vi "FGV_DataPackerQueueMetrics.vi"(7 "Enum":T1, 8 "Queue Size":i32, 9 "Elements bundled for serialisation":i32, 10 "# elements in queue":i32, 11 "Unique Banks to serialise":i32) -> (0 "Queue Size":i32, 1 "Elements bundled for serialisation":i32, 2 "# elements in queue":i32, 3 "Unique Banks to serialise":i32)   [LabVIEW 2018, in "feGEM DataPacker.lvlib"]
uses:
  Set_And_Get_Enum.ctl
  feGEM DataPacker.lvlib
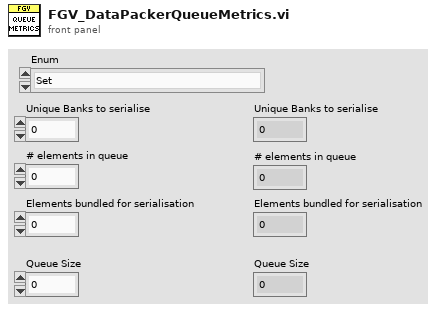
[diagram p1: front panel]
types:
  T1 = typedef "feGEM DataPacker.lvlib/Set_And_Get_Enum.ctl" = enum16{"Set", "Get"}
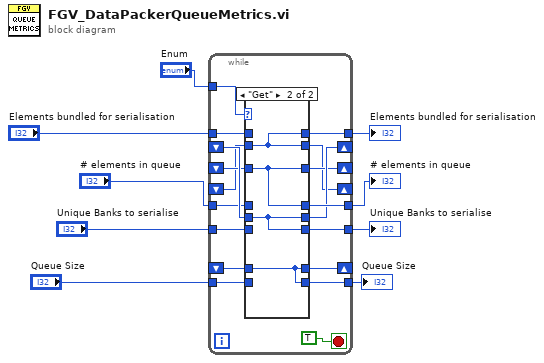
[diagram p0: block diagram]
diagram:
  n1 = while {
    tunnel: "Unique Banks to serialise" -> [w25]
    tunnel: "Enum" -> [w26]
    tunnel: [w24] -> w8
    shift-right: [w23] -> _
    shift-left: _ -> [w21]
    shift-right: [w22] -> _
    shift-left: _ -> [w20]
    tunnel: [w19] -> w9
    tunnel: [w18] -> w7
    shift-right: [w17] -> _
    shift-left: _ -> [w16]
    tunnel: "# elements in queue" -> [w14]
    tunnel: "Elements bundled for serialisation" -> [w15]
    tunnel: "Queue Size" -> [w13]
    tunnel: [w12] -> w1
    shift-right: [w11] -> _
    shift-left: _ -> [w10]
    stop <- TRUE stop-if-true
    n2 = case shown="\"Get\"" w26 {
      tunnel: w25 -> [w29 _]
      tunnel: [w30 w34] -> w24
      tunnel: [w29 w33] -> w23
      tunnel: [w30 w34] -> w22
      tunnel: w21 -> [_ w33]
      tunnel: w20 -> [_ w34]
      tunnel: [w29 w33] -> w19
      tunnel: [w31 w35] -> w18
      tunnel: w16 -> [_ w35]
      tunnel: [w31 w35] -> w17
      tunnel: w15 -> [w31 _]
      tunnel: w14 -> [w30 _]
      tunnel: w13 -> [w28 _]
      tunnel: [w28 w32] -> w12
      tunnel: [w28 w32] -> w11
      tunnel: w10 -> [_ w32]
      frame "Set", Default {
      }
      frame "Get" {
      }
    }
  }
  "# elements in queue" <- w8
  "Elements bundled for serialisation" <- w7
  "Unique Banks to serialise" <- w9
  "Queue Size" <- w1
